vi "Write Analog.vi"(8 "error in (no error)":errorcluster, 10 "Params":variant, 11 "NI Analog Output in":refnum<class "NI Analog Output.lvclass">) -> (0 "error out":errorcluster, 3 "NI Analog Output out":refnum<class "NI Analog Output.lvclass">)   [LabVIEW 2020, in "NI DAQmx.lvlib" / "NI Analog Output.lvclass"]
uses:
  NI Analog Output.lvclass
  D:/WSGitHub/RTFWK/Realization/NI DAQmx Base/NI DAQmx Base.lvclass
  <vilib>/DAQmx/write.llb/DAQmx Write (Analog DBL 1Chan 1Samp).vi
  <vilib>/DAQmx/write.llb/DAQmx Write (Analog 1D DBL 1Chan NSamp).vi
  <vilib>/DAQmx/write.llb/DAQmx Write (Analog 2D DBL NChan NSamp).vi
  <vilib>/DAQmx/write.llb/DAQmx Write (Analog 1D DBL NChan 1Samp).vi
  <vilib>/DAQmx/miscellaneous.llb/DAQmx Fill In Error Info.vi
  <resource>/objmgr/daqmx.rc
  <vilib>/Utility/Data Type/NI_Data Type.lvlib
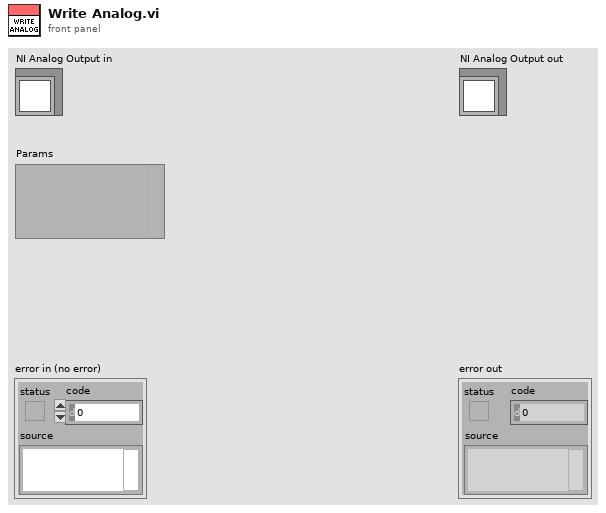
[diagram p1: front panel]
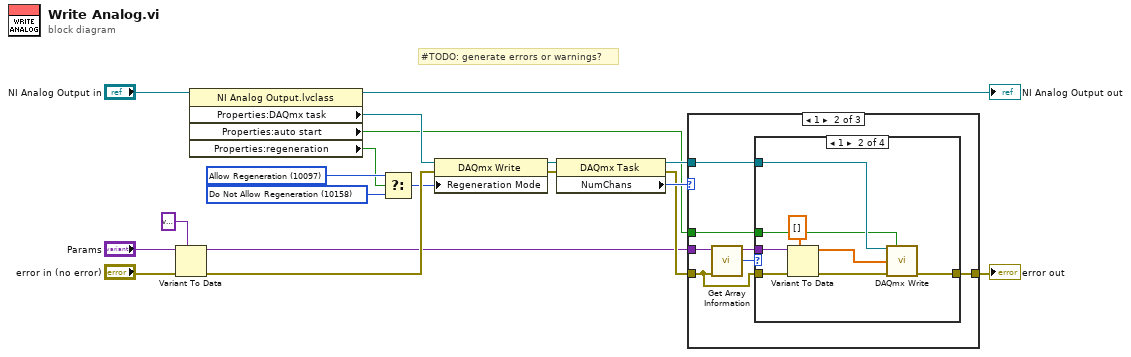
[diagram p0: block diagram]
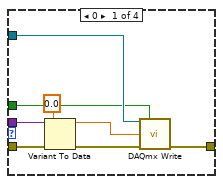
[diagram p3: hidden frame]
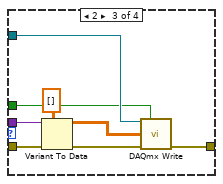
[diagram p4: hidden frame]
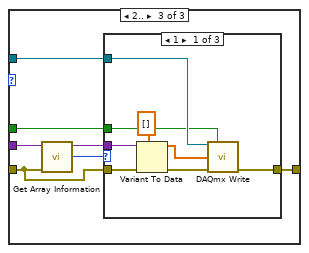
[diagram p6: hidden frame]
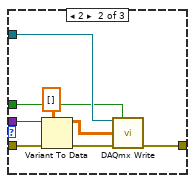
[diagram p7: hidden frame]
diagram:
  w6 = 10158 items=["Allow Regeneration"=10097, "Do Not Allow Regeneration"=10158] ("RegenMode")
  w7 = 10097 items=["Allow Regeneration"=10097, "Do Not Allow Regeneration"=10158] ("RegenMode")
  # "#TODO: generate errors or warnings?"
  n1 = Variant To Data(error in="error in (no error)", type=variant, Variant="Params") -> (data=w3:variant, error out=w10:errorcluster)
  n2 = property class="NI Analog Output.lvclass"(reference="NI Analog Output in") -> (reference out=→"NI Analog Output out":refnum<class "NI Analog Output.lvclass">, "Properties:DAQmx task"=w11:refnum<k21>, "Properties:auto start"=w1:bool, "Properties:regeneration"=w2:bool)  [unwired: 1 in, 1 out]
  n3 = Select(t=w7, s=w2, f=w6) -> (s? t:f=w8:i32)
  n4 = property class="DAQmx Write"(reference=w11, error in=w10, "Regeneration Mode"=w8) -> (reference out=w13:refnum<k21>, error out=w12:errorcluster)
  n5 = property class="DAQmx Task"(reference=w13, error in=w12) -> (reference out=w15:refnum<k21>, error out=w9:errorcluster, "NumChans"=w14:u32)
  n6 = case shown="1" w14 {
    tunnel: [w20 w26 w57] -> w16
    tunnel: w9 -> [w20 w21 w52]
    tunnel: w3 -> [_ w23 w54]
    tunnel: w15 -> [_ w25 w56]
    tunnel: w1 -> [_ w22 w53]
    frame 0, Default {
      # "no channels in task"
    }
    frame 1 {
      n7 = call <vilib>:"Get Array Information.vi"("error in (no error)"=w21, "variant"=w23) -> ("number of dimensions"=w24:i32)  [unwired: 6 in, 3 out]
      n8 = case shown="1" w24 {
        tunnel: [w31 w42 w50 w51] -> w26
        tunnel: w25 -> [w30 w40 w48 _]
        tunnel: w23 -> [w29 w37 w45 _]
        tunnel: w22 -> [w28 w36 w44 _]
        tunnel: w21 -> [w27 w35 w43 w51]
        frame 0 {
          n9 = Variant To Data(error in=w27, type=0.0 ("Numeric"), Variant=w29) -> (data=w33:dbl, error out=w34:errorcluster)
          n10 = call-poly <vilib>:"DAQmx Write.vi"("task/channels in"=w30, "auto start"=w28, "data"=w33, "error in"=w34) -> ("error out"=w31:errorcluster)  [unwired: 9 in, 2 out]
        }
        frame 1 {
          n11 = Variant To Data(error in=w35, type=dbl[] [] ("Numeric"), Variant=w37) -> (data=w39:dbl[], error out=w41:errorcluster)
          n12 = call-poly <vilib>:"DAQmx Write.vi"("task/channels in"=w40, "auto start"=w36, "data"=w39, "error in"=w41) -> ("error out"=w42:errorcluster)  [unwired: 9 in, 2 out]
        }
        frame 2 {
          n13 = Variant To Data(error in=w43, type=dbl[][] [] ("Numeric"), Variant=w45) -> (data=w47:dbl[][], error out=w49:errorcluster)
          n14 = call-poly <vilib>:"DAQmx Write.vi"("task/channels in"=w48, "auto start"=w44, "data"=w47, "error in"=w49) -> ("error out"=w50:errorcluster)  [unwired: 9 in, 2 out]
        }
        frame Default {
          # "invalid data type"
        }
      }
    }
    frame 2.. {
      n15 = call <vilib>:"Get Array Information.vi"("error in (no error)"=w52, "variant"=w54) -> ("number of dimensions"=w55:i32)  [unwired: 6 in, 3 out]
      n16 = case shown="1" w55 {
        tunnel: [w65 w73 w74] -> w57
        tunnel: w56 -> [w63 w71 _]
        tunnel: w54 -> [w59 w67 _]
        tunnel: w53 -> [w60 w68 _]
        tunnel: w52 -> [w58 w66 w74]
        frame 1 {
          n17 = Variant To Data(error in=w58, type=dbl[] [] ("Numeric"), Variant=w59) -> (data=w62:dbl[], error out=w64:errorcluster)
          n18 = call-poly <vilib>:"DAQmx Write.vi"("task/channels in"=w63, "auto start"=w60, "data"=w62, "error in"=w64) -> ("error out"=w65:errorcluster)  [unwired: 9 in, 2 out]
        }
        frame 2 {
          n19 = Variant To Data(error in=w66, type=dbl[][] [] ("Numeric"), Variant=w67) -> (data=w70:dbl[][], error out=w72:errorcluster)
          n20 = call-poly <vilib>:"DAQmx Write.vi"("task/channels in"=w71, "auto start"=w68, "data"=w70, "error in"=w72) -> ("error out"=w73:errorcluster)  [unwired: 9 in, 2 out]
        }
        frame Default {
        }
      }
    }
  }
  "error out" <- w16
